vi "solar_app ExeVersion.vi"() -> (1 "ExeVersion":string, 2 "ExePath":path, 5 "Run-Time System?":bool)   [LabVIEW 2018]
doc: "This returns the Executable path and version."
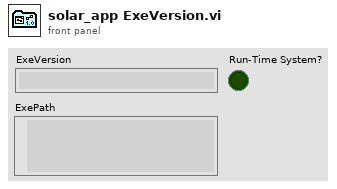
[diagram p1: front panel]
types:
  T1 = enum32{"invalid app kind", "Development System", "Run Time System", "Student Edition", "Embedded LabVIEW", "Evaluation", "Custom"}
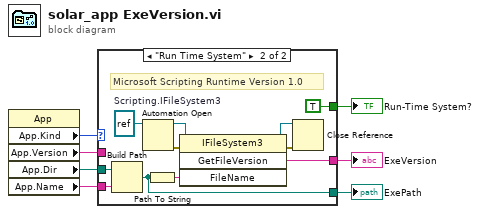
[diagram p0: block diagram]
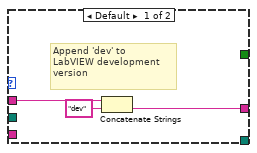
[diagram p2: hidden frame]
diagram:
  n1 = property class="App"() -> ("App.Kind"=w3:T1, "App.Version"=w4:string, "App.Dir"=w1:path, "App.Name"=w2:string)  [unwired: 2 in, 2 out]
  n2 = case shown="\"Run Time System\"" w3 {
    tunnel: w1 -> [_ w15]
    tunnel: w2 -> [_ w14]
    tunnel: [w8 w13] -> w7
    tunnel: w4 -> [w10 _]
    tunnel: [_ w12] -> w6
    tunnel: [_ TRUE] -> w5
    frame Default {
      # "Append 'dev' to\nLabVIEW development \nversion"
      n3 = Concatenate Strings(w10, "dev" ("string")) -> (w8:string)
    }
    frame "Run Time System" {
      w21 = refnum<k7> refnum  # Scripting.IFileSystem3
      # "Microsoft Scripting Runtime Version 1.0"
      n4 = Build Path(base path=w15, name or relative path=w14) -> (appended path=w12:path)
      n5 = Automation Open(Automation Refnum=w21) -> (Automation Refnum=w20:refnum<k7>, error out=w19:errorcluster)  [unwired: 1 in, 2 out]
      n6 = Path To String(path=w12) -> (string=w16:string)
      n7 = invoke class="IFileSystem3" method="GetFileVersion"(reference=w20, error in=w19, "FileName"=w16) -> (reference out=w18:refnum<k7>, error out=w17:errorcluster, "GetFileVersion"=w13:string)  [unwired: 1 in, 1 out]
      n8 = Close Reference(reference=w18, error in (no error)=w17) -> ()  [unwired: 1 out]
    }
  }
  "ExeVersion" <- w7
  "ExePath" <- w6
  "Run-Time System?" <- w5
